vi "8888888888888888888888888.vi"   [LabVIEW 2018]
uses:
  <vilib>/Instr/_visa.llb/VISA Configure Serial Port (Instr).vi
  Subvi/Global.vi
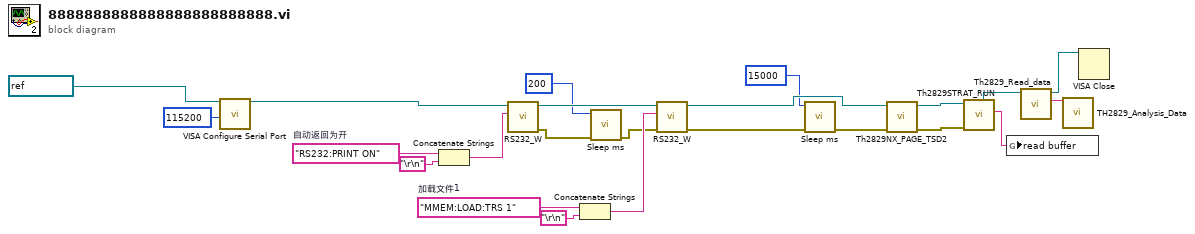
[diagram p0: block diagram]
diagram:
  w12 = "RS232:PRINT ON"  # 自动返回为开
  w10 = "MMEM:LOAD:TRS 1"  # 加载文件1
  n1 = call-poly "VISA Configure Serial Port"("VISA resource name"=refnum<visa-resource-name> "COM3", "baud rate (9600)"=u32 115200) -> ("VISA resource name out"=w16:refnum<visa-resource-name>)  [unwired: 12 in, 1 out]
  n2 = Concatenate Strings(w12, "\r\n") -> (w7:string)
  n3 = call "RS232_W.vi"("CMD"=w7, "VISA资源名称"=w16) -> ("error out"=w3:errorcluster, "VISA资源名称输出"=w6:refnum<visa-resource-name>)  [unwired: 7 in, 1 out]
  n4 = Concatenate Strings(w10, "\r\n") -> (w9:string)
  n5 = call "Sleep ms.vi"("error in (no error)"=w3, "等待时间（毫秒）"=u32 200) -> ("error out"=w2:errorcluster)  [unwired: 9 in]
  n6 = call "RS232_W.vi"("error in (no error)"=w2, "CMD"=w9, "VISA资源名称"=w6) -> ("error out"=w5:errorcluster, "VISA资源名称输出"=w14:refnum<visa-resource-name>)  [unwired: 6 in, 1 out]
  n7 = call "Sleep ms.vi"("error in (no error)"=w5, "等待时间（毫秒）"=u32 15000) -> ("error out"=w13:errorcluster)  [unwired: 9 in]
  n8 = call "Th2829NX_PAGE_TSD2.vi"("错误输入（无错误）"=w13, "VISA资源名称"=w14) -> ("error out"=w19:errorcluster, "VISA资源名称输出"=w21:refnum<visa-resource-name>)  [unwired: 8 in]
  n9 = call "Th2829STRAT_RUN.vi"("错误输入（无错误）"=w19, "VISA资源名称"=w21) -> ("read buffer"=w20:string, "VISA资源名称 2"=w23:refnum<visa-resource-name>)  [unwired: 6 in, 2 out]
  n10 = global write "Global.vi" "read buffer"(w20) -> ()
  n11 = call "Th2829_Read_data.vi"("VISA资源名称"=w23) -> ("读取缓冲区"=w22:string, "VISA资源名称 2"=w17:refnum<visa-resource-name>)  [unwired: 9 in]
  n12 = call "TH2829_Analysis_Data.vi"("字符串"=w22) -> ()  [unwired: 15 in, 4 out]
  n13 = VISA Close(VISA resource name=w17) -> ()  [unwired: 1 in, 1 out]
